vi "Set Parameters GUI.vi"(8 "error in (no error)":errorcluster, 11 "Lakeshore 331 in":refnum<class "Lakeshore 331.lvclass">) -> (0 "error out":errorcluster, 3 "Lakeshore 331 out":refnum<class "Lakeshore 331.lvclass">)   [LabVIEW 2022 SP3, in "Lakeshore 331.lvclass"]
uses:
  Lakeshore 331.lvclass
  Lakeshore 331.lvclass/Lakeshore 331.ctl
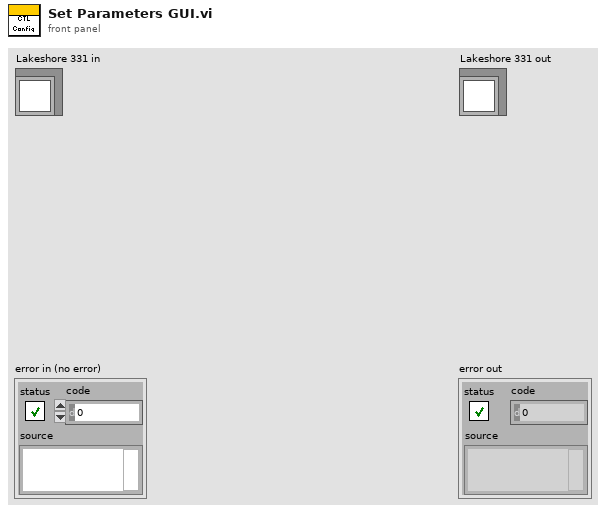
[diagram p1: front panel]
types:
  T1 = typedef "Lakeshore 331.lvclass/Lakeshore 331 Parameters.ctl" = cluster{"Mode":u16, "Setpoint":dbl, "Manual Power (%)":dbl, "Control Parameters":cluster{"P":dbl, "I":dbl, "D":u16}}
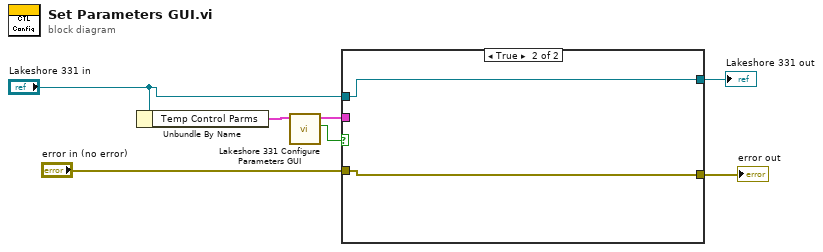
[diagram p0: block diagram]
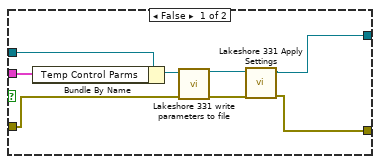
[diagram p2: hidden frame]
diagram:
  n1 = Unbundle By Name("Lakeshore 331 in") -> ("Temp Control Parms"=w7:T1)
  n2 = call "Lakeshore 331 Configure Parameters GUI.vi"("Temp Control Parms"=w7) -> ("Cancelled"=w6:bool, "Temp Control Parms out"=w5:T1)  [unwired: 9 in]
  n3 = case shown="True" w6 {
    tunnel: w5 -> [w14 _]
    tunnel: "Lakeshore 331 in" -> [w15 w17]
    tunnel: [w10 w17] -> w3
    tunnel: [w9 w16] -> w2
    tunnel: "error in (no error)" -> [w8 w16]
    frame False {
      n4 = Bundle By Name(cluster=w15, "Temp Control Parms"=w14) -> (w13:refnum<class "Lakeshore 331.lvclass">)
      n5 = call "Lakeshore 331 write parameters to file.vi"("error in (no error)"=w8, "Lakeshore 331 in"=w13) -> ("error out"=w12:errorcluster, "Lakeshore 331 out"=w11:refnum<class "Lakeshore 331.lvclass">)  [unwired: 8 in]
      n6 = call "Lakeshore 331 Apply Settings.vi"("error in (no error)"=w12, "Lakeshore 331 in"=w11) -> ("error out"=w9:errorcluster, "Lakeshore 331 out"=w10:refnum<class "Lakeshore 331.lvclass">)  [unwired: 8 in]
    }
    frame True {
    }
  }
  "error out" <- w2
  "Lakeshore 331 out" <- w3
